vi "Joystick Sensitivity.vi"(9 "b":dbl, 10 "a":dbl, 11 "x":dbl) -> (3 "y":dbl)   [LabVIEW 2014]
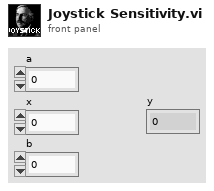
[diagram p1: front panel]
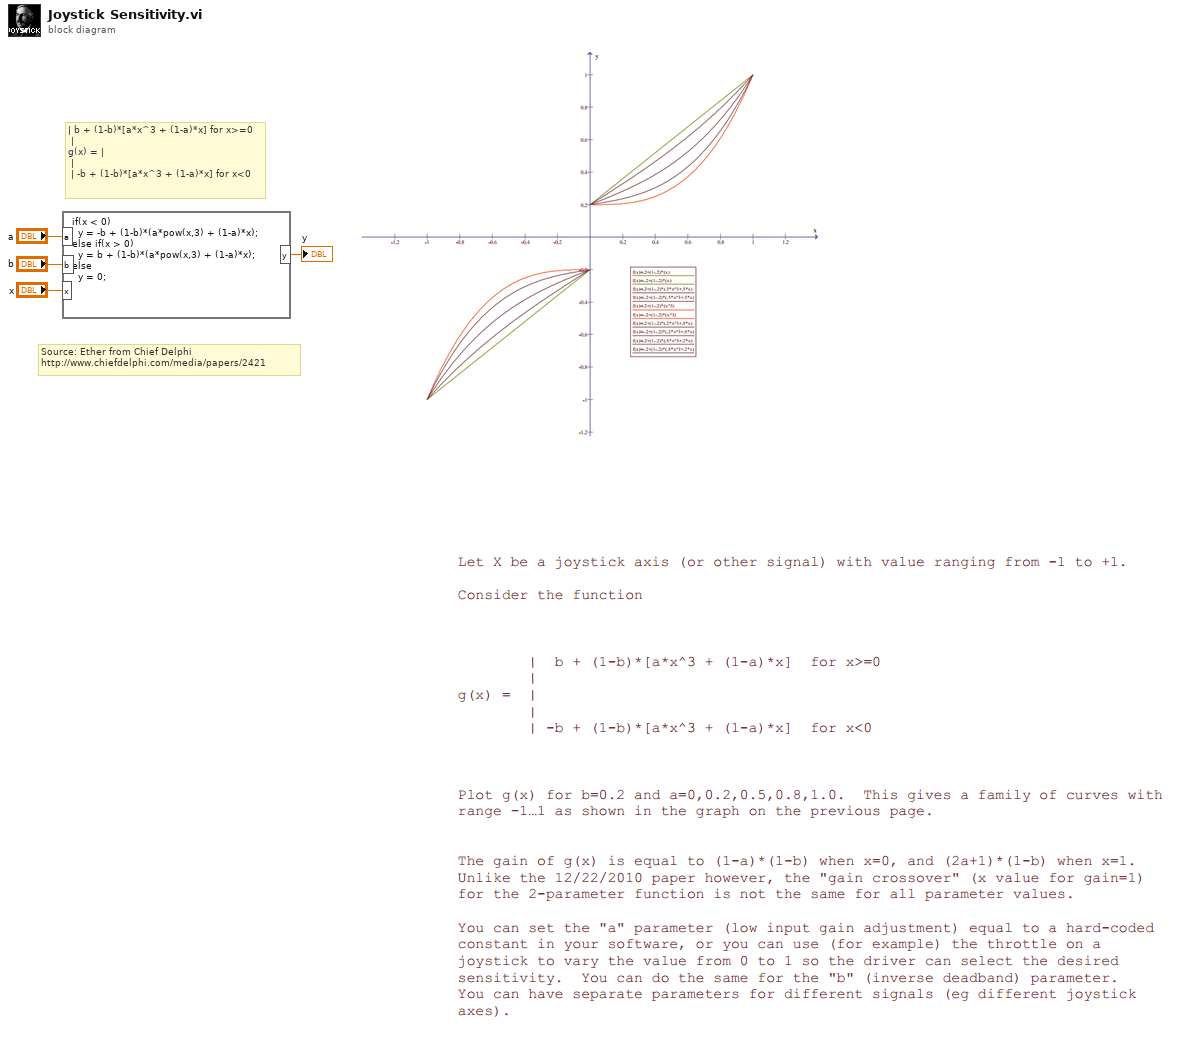
[diagram p0: block diagram]
diagram:
  # "Source: Ether from Chief Delphi\nhttp://www.chiefdelphi.com/media/papers/2421"
  # "| b + (1-b)*[a*x^3 + (1-a)*x] for x>=0\n |\ng(x) = |\n |\n | -b + (1-b)*[a*x^3 + (1-a)*x] for x<0"
  n1 = formula code="if(x < 0)\n  y = -b + (1-b)*(a*pow(x,3) + (1-a)*x);\nelse if(x > 0)\n  y = b + (1-b)*(a*pow(x,3) + (1-a)*x);\nelse\n  y = 0;"("a"="a", "x"="x", "b"="b") -> ("y"=→"y":dbl)
